vi "LSX Get Encoder Active.vi"(8 "error in (no error)":errorcluster, 10 "plFlags":i32, 11 "lLSID":i32) -> (0 "error out":errorcluster, 2 "plFlags out":i32, 3 "function return":i32)   [LabVIEW 2018, in "Tango.lvlib"]
doc: "TANGOAPI int TANGOCALL LSX_GetEncoderActive (int lLSID, int *plFlags);"
uses:
  <userlib>/Tango/Tango.lvlib
  <userlib>/Tango/Tango_DLL.dll
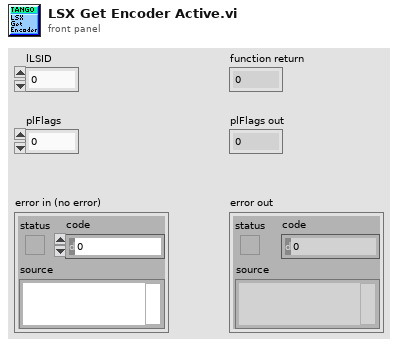
[diagram p1: front panel]
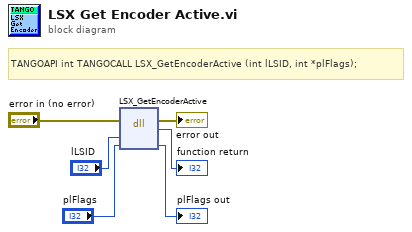
[diagram p0: block diagram]
diagram:
  # "TANGOAPI int TANGOCALL LSX_GetEncoderActive (int lLSID, int *plFlags);"
  n1 = dll-call lib="C:/Program Files (x86)/National Instruments/LabVIEW 2018/user.lib/Tango/Tango_DLL.*" fn="LSX_GetEncoderActive"(error in="error in (no error)", "lLSID"="lLSID", "plFlags"="plFlags") -> (error out=→"error out":errorcluster, →"function return":i32, "plFlags"=→"plFlags out":i32)  [unwired: 3 in, 1 out]
